vi "IOP Sensor Calibration.vi"() -> (3 "IOP Output [mmHg]":dbl[](array[numeric]))   [LabVIEW 2016]
uses:
  <vilib>/Platform/TimedLoop/XDataNode/timing_clust.ctl
  <vilib>/Platform/TimedLoop/XDataNode/nitl_modes.ctl
  <vilib>/Platform/TimedLoop/XDataNode/wakeup.ctl
  <vilib>/FPGAPlugInAG/PXI-7833R/niLvFpga_Open_PXI-7833R.vi
  <vilib>/Utility/error.llb/Error Cluster From Error Code.vi
  <vilib>/rvi/errors/niLvFpgaAdjustHostInterfaceError.vi
  <vilib>/rvi/interface/nirviOpenFPGA/nirviOpenFPGA.xnode
  FPGA Bitfiles/PhantomControlPI_FPGATarget_QuadCtr2_E2412E44.lvbitx
  IRISS_FPGA_IO.vi
  <vilib>/platform/TimedLoop/XDataNode/XDataNode.xnode
  <vilib>/rvi/interface/nirviReadWriteControl/nirviReadWriteControl.xnode
  <vilib>/Platform/TimedLoop/XDataNode/XDNodeRunTimeDep.lvlib
  NiFpgaLv.dll
panel:
  in  "Vacuum Cmd":sgl min=0 max=600
  in  "Irrigation Height":i32 min=0 max=90 step=5
  in  "Program Stop":bool
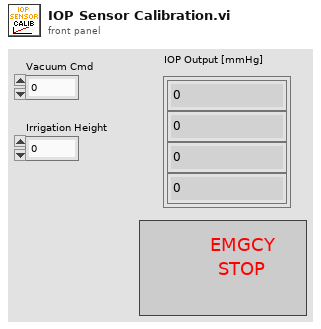
[diagram p1: front panel]
types:
  T1 = typedef "XDNodeRunTimeDep.lvlib/timing_clust.ctl" = cluster{"Expected End [f-1]":u64, "Actual End [f-1]":u64, "Finished Late? [f-1]":bool, "Expected End [i-1]":u64, "Actual End [i-1]":u64, "Finished Late? [i-1]":bool, "Expected Start [i]":u64, "Actual Start [i]":u64, "Expected Start [f]":u64, "Actual Start [f]":u64, "Source Name":string, "Structure Name":string, "Period":i64, "Deadline":i64, "Offset":i64, "Start":i64, "Priority":i32, "Timeout":i32, "Mode":T2, "Wakeup Reason":T3, "Error":errorcluster, "Source Type":string, "Secondary Source Type":string, "Global End Time":u64, "Global Start Time":u64, "Frame Duration":u64, "Iteration Duration":u64, "Assigned CPU":i32, "I/O Scan Engine Mode":u32}
  T2 = typedef "XDNodeRunTimeDep.lvlib/nitl_modes.ctl" = enum32{"No Change", "Process missed periods, maintain original phase", "Discard missed periods, maintain original phase", "Process missed periods, ignore original phase", "Discard missed periods, ignore original phase"}
  T3 = typedef "XDNodeRunTimeDep.lvlib/wakeup.ctl" = enum32{"Normal", "Aborted", "Asynchronous wakeup", "Timing source error", "Timed loop error", "Timeout"}
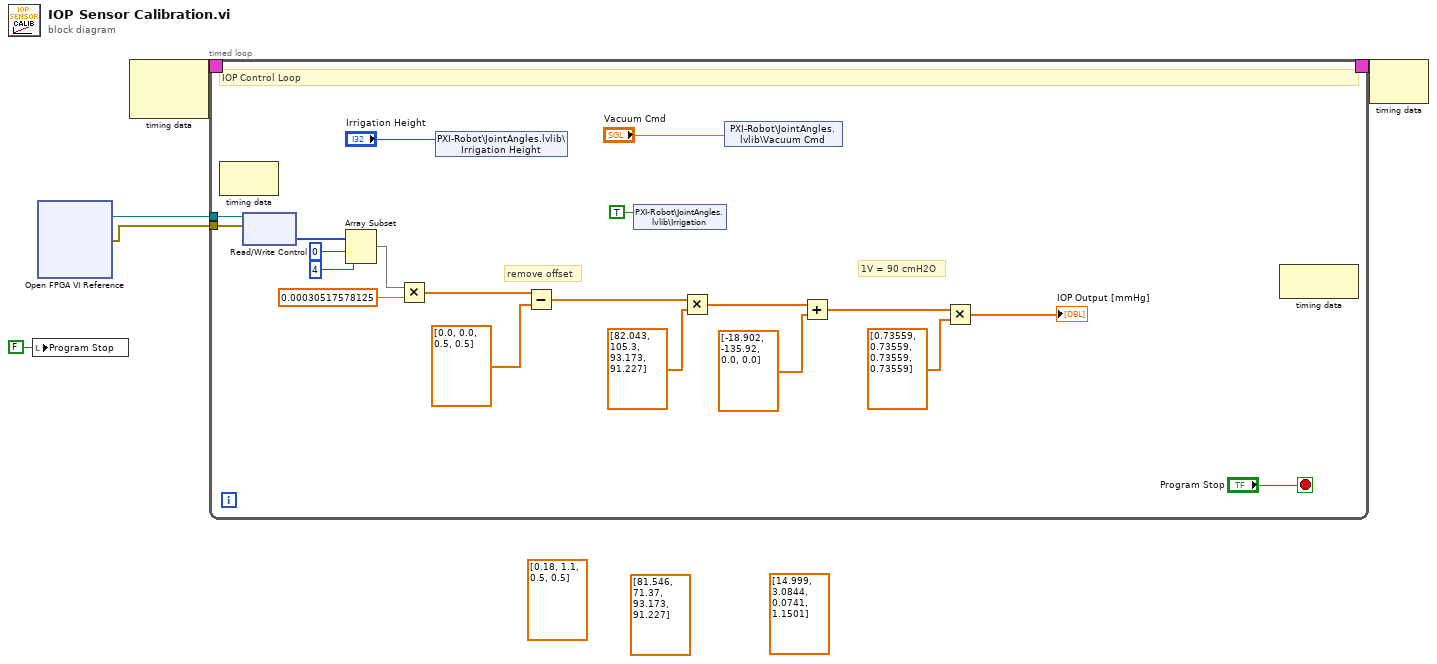
[diagram p0: block diagram]
diagram:
  (unwired) dbl[] [0.18, 1.1, 0.5, 0.5]
  (unwired) dbl[] [81.546, 71.37, 93.173, 91.227]
  (unwired) dbl[] [14.999, 3.0844, 0.0741, 1.1501]
  n1 = local write "Program Stop"(FALSE ("Program Stop")) -> ()
  n2 = xnode "Open FPGA VI Reference"() -> ("FPGA VI Reference Out"=w3:refnum<k20>, "error out"=w2:errorcluster)  [unwired: 2 in]
  n3 = node-c288 ("Input Node")() -> (w5:T1)  [unwired: 2 in]
  n4 = timed-loop {
    timing: w5 -> [_]
    timing-out: [_] -> w4
    tunnel: w3 -> [w20]
    tunnel: w2 -> [w19]
    stop <- "Program Stop" stop-if-true
    # "remove offset"
    # "1V = 90 cmH2O"
    # "IOP Control Loop"
    n5 = node-c288() -> ()  [unwired: 1 in, 1 out]
    n6 = xnode "Read/Write Control"("FPGA VI Reference In"=w20, "error in"=w19) -> ("AI"=w21:i16[])  [unwired: 2 out]
    n7 = Array Subset(array=w21, index=0, length=4) -> (w25:i16[])
    n8 = Multiply(x=w25, y=0.00030517578125) -> (x*y=w10:dbl[])
    n9 = shared-variable "PXI-Robot\\JointAngles.lvlib\\Irrigation Height"("Irrigation Height") -> ()  [unwired: 1 in, 1 out]
    n10 = Subtract(x=w10, y=dbl[] [0.0, 0.0, 0.5, 0.5]) -> (x-y=w13:dbl[])
    n11 = shared-variable "PXI-Robot\\JointAngles.lvlib\\Irrigation"(TRUE ("Irrigation")) -> ()  [unwired: 1 in, 1 out]
    n12 = Multiply(x=w13, y=dbl[] [82.043, 105.3, 93.173, 91.227]) -> (x*y=w15:dbl[])
    n13 = shared-variable "PXI-Robot\\JointAngles.lvlib\\Vacuum Cmd"("Vacuum Cmd") -> ()  [unwired: 1 in, 1 out]
    n14 = Add(x=w15, y=dbl[] [-18.902, -135.92, 0.0, 0.0]) -> (x+y=w16:dbl[])
    n15 = Multiply(x=w16, y=dbl[] [0.73559, 0.73559, 0.73559, 0.73559]) -> (x*y=→"IOP Output [mmHg]":dbl[])
    n16 = node-c288() -> ()  [unwired: 1 in, 1 out]
  }
  n17 = node-c288(w4) -> ()  [unwired: 1 out]
